vi "AddStartProcess.vi"(8 "error in (no error)":errorcluster, 11 "AppContextIn":T1={"VIRefToProcessTemplate"=refnum, "VIRefToThisVI"=refnum, "ProcessesList"=[], "VIRefToEnumProcess"=refnum, "VIRefTogetProcessViPath"=refnum, "ProcessManagement"={"EnumProcessState"=enum."Create process", "ProcessName"="", "PathToProcess"=path ""}, "VIRefToSetup"=refnum, "VIRefToStartProcess"=refnum, "ProcessConfig"={"File Path Control"=path "", "Timeout"=0.0, "viInitString"="", "State"=enum."Closed"}}) -> (0 "error out":errorcluster, 3 "AppContextOut":T1={"VIRefToProcessTemplate"=refnum, "VIRefToThisVI"=refnum, "ProcessesList"=[], "VIRefToEnumProcess"=refnum, "VIRefTogetProcessViPath"=refnum, "ProcessManagement"={"EnumProcessState"=enum."Create process", "ProcessName"="", "PathToProcess"=path ""}, "VIRefToSetup"=refnum, "VIRefToStartProcess"=refnum, "ProcessConfig"={"File Path Control"=path "", "Timeout"=0.0, "viInitString"="", "State"=enum."Closed"}})   [LabVIEW 2013]
uses:
  Ctl/AppContext.ctl
  Ctl/EnumProcessState.ctl
  050 - CONFIG/20 - ExternalProcesses/paramsExternalProcesses.ctl
  Class/Process/Process.lvclass
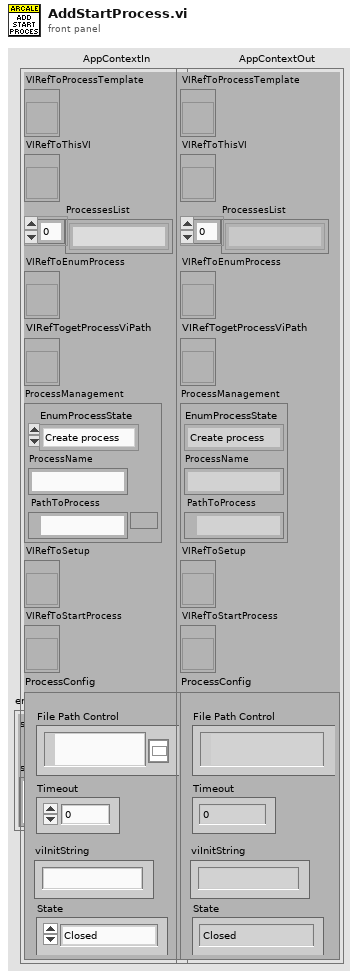
[diagram p1: front panel]
types:
  T1 = typedef "AppContext.ctl" = cluster{"VIRefToProcessTemplate":refnum<vi>, "VIRefToThisVI":refnum<vi>, "ProcessesList":string[], "VIRefToEnumProcess":refnum<vi>, "VIRefTogetProcessViPath":refnum<vi>, "ProcessManagement":cluster{"EnumProcessState":T2, "ProcessName":string, "PathToProcess":path}, "VIRefToSetup":refnum<vi>, "VIRefToStartProcess":refnum<vi>, "ProcessConfig":T3}
  T2 = typedef "EnumProcessState.ctl" = enum16{"Create process", "Delete process"}
  T3 = typedef "paramsExternalProcesses.ctl" = cluster{"File Path Control":path, "Timeout":dbl, "viInitString":string, "State":enum32{"Invalid", "Standard", "Closed", "Hidden", "Minimized", "Maximized"}}
  T4 = typedef "LVPositionTypeDef.ctl" = cluster{"Left":i32, "Top":i32}
  T5 = typedef "LVPointTypeDef.ctl" = cluster{"Horizontal":i16, "Vertical":i16}
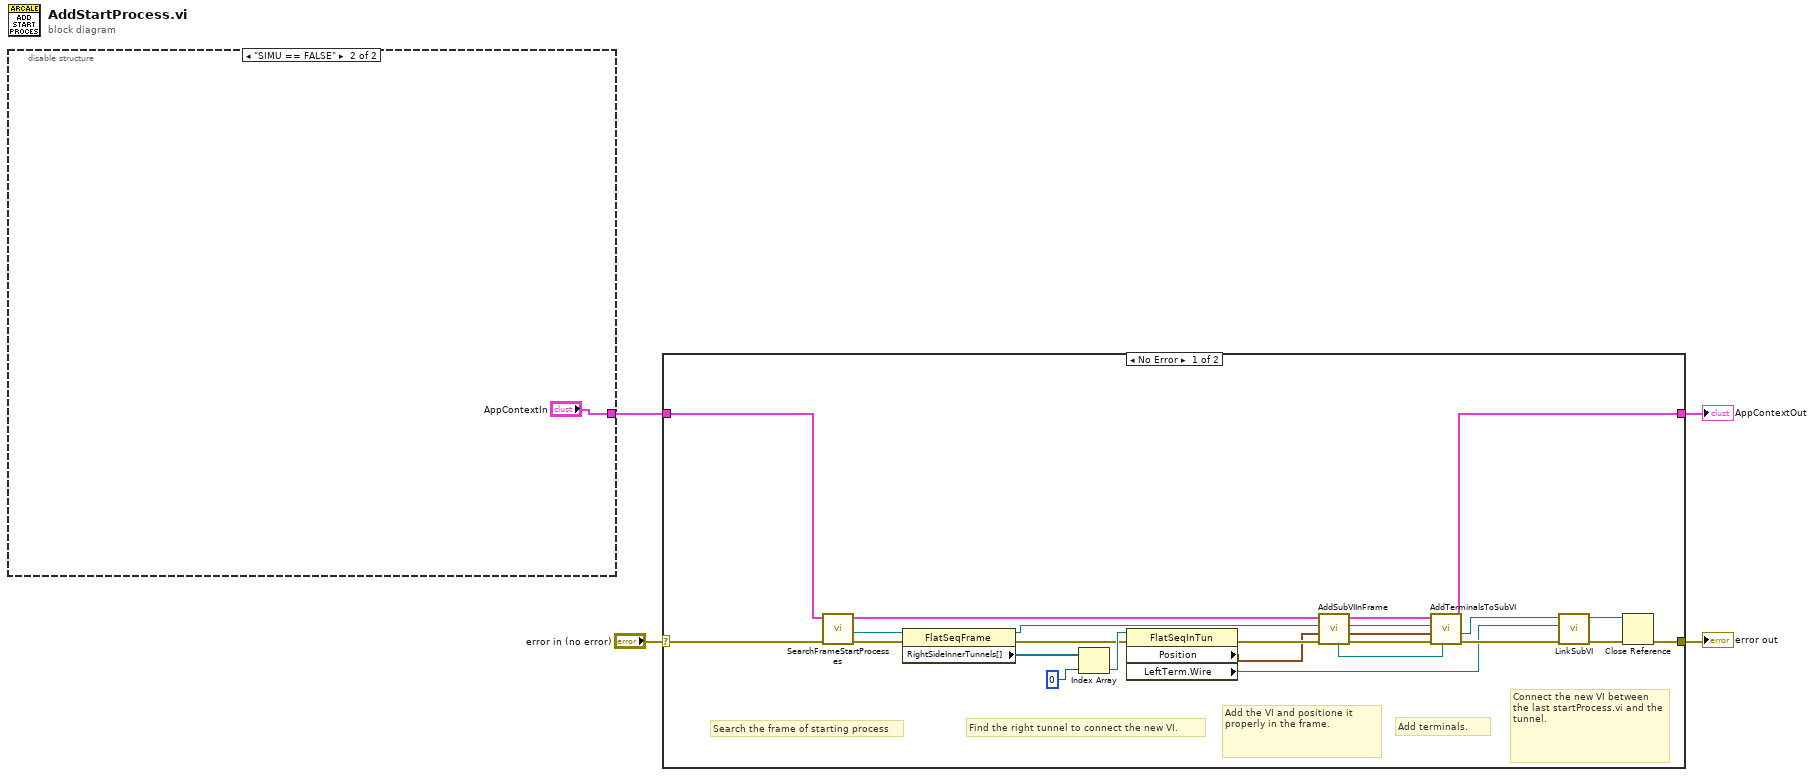
[diagram p0: block diagram]
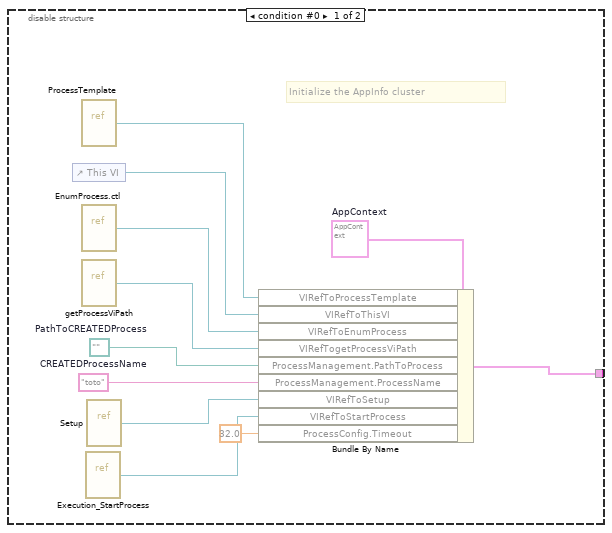
[diagram p2: hidden frame]
diagram:
  n1 = disable-structure shown="\"SIMU == FALSE\"" {
    disable-tunnel: [w6 "AppContextIn"] -> w1
    frame condition #0 {
      w9 = T1 {"VIRefToProcessTemplate"=refnum, "VIRefToThisVI"=refnum, "ProcessesList"=[], "VIRefToEnumProcess"=refnum, "VIRefTogetProcessViPath"=refnum, "ProcessManagement"={"EnumProcessState"=enum."Create process", "ProcessName"="", "PathToProcess"=path ""}, "VIRefToSetup"=refnum, "VIRefToStartProcess"=refnum, "ProcessConfig"={"File Path Control"=path "", "Timeout"=0.0, "viInitString"="", "State"=enum."Invalid"}}  # AppContext
      w10 = "toto"  # CREATEDProcessName
      w11 = path ""  # PathToCREATEDProcess
      # "Initialize the AppInfo cluster"
      n2 = control-ref of="This VI"() -> (w14:refnum<vi>)
      n3 = vi-ref "ProcessTemplate.vi"() -> (w15:refnum<vi>)
      n4 = vi-ref "EnumProcess.ctl"() -> (w13:refnum<vi>)
      n5 = vi-ref "getProcessViPath.vi"() -> (w12:refnum<vi>)
      n6 = vi-ref "Execution_StartProcess.vi"() -> (w7:refnum<vi>)
      n7 = vi-ref "Setup.vi"() -> (w8:refnum<vi>)
      n8 = Bundle By Name(cluster=w9, "VIRefToProcessTemplate"=w15, "VIRefToThisVI"=w14, "VIRefToEnumProcess"=w13, "VIRefTogetProcessViPath"=w12, "ProcessManagement.PathToProcess"=w11, "ProcessManagement.ProcessName"=w10, "VIRefToSetup"=w8, "VIRefToStartProcess"=w7, "ProcessConfig.Timeout"=32.0 ("ProcessManagement.Timeout")) -> (w6:T1)
    }
    frame condition #1 (active) {
    }
  }
  n9 = case shown="No Error" "error in (no error)" {
    selector: "error in (no error)" -> [w35 w42]
    tunnel: [w18 w42] -> w3
    tunnel: [w22 w41] -> w2
    tunnel: w1 -> [w32 w41]
    frame No Error {
      # "Connect the new VI between the last startProcess.vi and the tunnel."
      # "Search the frame of starting process"
      # "Add terminals."
      # "Find the right tunnel to connect the new VI."
      # "Add the VI and positione it properly in the frame."
      n10 = call "SearchFrameStartProcesses.vi"("error in (no error)"=w35, "AppContextIn"=w32) -> ("error out"=w34:errorcluster, "FlatSequenceFrame out"=w33:refnum<vi>, "AppContextOut"=w29:T1)  [unwired: 7 in]
      n11 = property class="FlatSeqFrame"(reference=w33, error in=w34) -> (reference out=w28:refnum<vi>, error out=w37:errorcluster, "RightSideInnerTunnels[]"=w39:refnum<vi>[])
      n12 = Index Array(array=w39, index=0) -> (element=w38:refnum<vi>)
      n13 = property class="FlatSeqInTun"(reference=w38, error in=w37) -> (error out=w36:errorcluster, "Position"=w21:T4, "LeftTerm.Wire"=w20:refnum<vi>)  [unwired: 1 out]
      n14 = call "AddSubVIInFrame.vi"("error in (no error)"=w36, "RightInTunnelPosition"=w21, "SeqFrameRefnumIn"=w28, "AppContextIn"=w29) -> ("error out"=w30:errorcluster, "locationVIAdded"=w26:T5, "SeqFrameRefnumOut"=w27:refnum<vi>, "AppContextOut"=w23:T1, "VIaddedRefnum"=w25:refnum<vi>)  [unwired: 3 in]
      n15 = call "AddTerminalsToSubVI.vi"("SubVIRefnum In"=w25, "error in (no error)"=w30, "locationVIAdded"=w26, "FrameRefnum"=w27, "AppContextIn"=w23) -> ("error out"=w24:errorcluster, "SubVIRefnum Out"=w31:refnum<vi>, "AppContextOut"=w22:T1)  [unwired: 4 in]
      n16 = call "LinkSubVI.vi"("error in (no error)"=w24, "WireRef"=w20, "SubVIRef In"=w31) -> ("error out"=w19:errorcluster, "SubVIRef Out"=w17:refnum<vi>)  [unwired: 7 in]
      n17 = Close Reference(reference=w17, error in (no error)=w19) -> (error out=w18:errorcluster)
    }
    frame Error {
    }
  }
  "error out" <- w3
  "AppContextOut" <- w2
